vi "DownLoad LTC-20 Table V0.80.vi"(0 "LTC-20 GPIB":refnum<visa-resource-name>, 2 "Sensor Selection":u16(ring) items=["Old MultiSample30T", "New MultiSample Probe (heavy)", "TransmissionProbe 30T", "Double Sample 30T", "SingleSample 30T", "Voigt-6SampleProbe 20T", "Nurmikko30T Top-emission", "Wim MOKE Probe"], 5 "error in (no error)":errorcluster, 9 "Sensor BasePath":path=path "/Optics2mac/Thermometer Calibrations/ Optics") -> (14 "#Tables":i32, 16 "ManyCal?":string, 19 "error out":errorcluster)   [LabVIEW 2019]
uses:
  <vilib>/Utility/file.llb/Read From Spreadsheet File (DBL).vi
panel:
  in  "?":bool
  in  "?":bool
  out "Sensor":string=":CX1050X10903"
  out "Loading:":i32
  out "CalArray":string[](array[string])=["325.000,2.02480,", "320.000,2.02830,", "310.000,2.03560,", "300.000,2.04330,", "290.000,2.05150,", "280.000,2.05960,", "270.000,2.06840,", "260.000,2.07700,", "250.000,2.08660,", "240.000,2.09600,", "230.000,2.10620,", "220.000,2.11640,", "210.000,2.12740,", "200.000,2.13890,", "190.000,2.15060,", "180.000,2.16290,", "170.000,2.17600,", "160.000,2.18960,", "150.000,2.20390,", "140.000,2.21930,", "130.000,2.23510,", "120.000,2.25180,", "110.000,2.26960,", "100.000,2.28870,", "90.000,2.30910,", "80.000,2.33160,", "77.350,2.33790,", "75.000,2.34350,", "70.000,2.35620,", "60.000,2.38390,", "56.000,2.39580,", "54.000,2.40200,", "50.000,2.41500,", "46.000,2.42910,", "44.000,2.43630,", "40.000,2.45170,", "38.000,2.45980,", "36.000,2.46820,", "34.000,2.47700,", "32.000,2.48650,", "30.000,2.49610,", "28.000,2.50610,", "26.000,2.51680,", "24.000,2.52810,", "22.000,2.54030,", "20.000,2.55340,", "19.000,2.56040,", "18.000,2.56750,", "17.000,2.57510,", "16.000,2.58310,", "15.000,2.59170,", "14.000,2.60120,", "13.000,2.61050,", "12.000,2.62100,", "11.000,2.63250,", "10.000,2.64480,", "9.500,2.65150,", "9.000,2.65880,", "8.500,2.66660,", "8.000,2.67440,", "7.500,2.68330,", "7.000,2.69270,", "6.500,2.70230,", "6.000,2.71370,", "5.800,2.71840,", "5.400,2.72870,", "5.000,2.73950,", "4.600,2.75160,", "4.200,2.76480,", "4.000,2.77230,", "3.900,2.77610,", "3.800,2.78000,", "3.700,2.78390,", "3.600,2.78810,", "3.500,2.79240,", "3.400,2.79700,", "3.300,2.80160,", "3.200,2.80650,", "3.100,2.81150,", "3.000,2.81660,", "2.900,2.82200,", "2.800,2.82780,", "2.700,2.83370,", "2.600,2.84000,", "2.500,2.84660,", "2.400,2.85350,", "2.300,2.86120,", "2.200,2.86870,", "2.100,2.87700,", "2.000,2.88560,", "1.900,2.89500,", "1.800,2.90520,", "1.700,2.91630,", "1.600,2.92920,", "1.500,2.94380,", "1.400,2.96020,", "1.300,2.97870,"]
  out "CharMatch":string="SCALT4,2,0,OptCernoxX02158,-1.0,"
  out "TempData":sgl[](array[numeric])=[325.0, 320.0, 310.0, 300.0, 290.0, 280.0, 270.0, 260.0, 250.0, 240.0, 230.0, 220.0, 210.0, 200.0, 190.0, 180.0, 170.0, 160.0, 150.0, 140.0, 130.0, 120.0, 110.0, 100.0, 90.0, 80.0, 77.35, 75.0, 70.0, 60.0, 56.0, 54.0, 50.0, 46.0, 44.0, 40.0, 38.0, 36.0, 34.0, 32.0, 30.0, 28.0, 26.0, 24.0, 22.0, 20.0, 19.0, 18.0, 17.0, 16.0, 15.0, 14.0, 13.0, 12.0, 11.0, 10.0, 9.5, 9.0, 8.5, 8.0, 7.5, 7.0, 6.5, 6.0, 5.8, 5.4, 5.0, 4.6, 4.2, 4.0, 3.9, 3.8, 3.7, 3.6, 3.5, 3.4, 3.3, 3.2, 3.1, 3.0, 2.9, 2.8, 2.7, 2.6, 2.5, 2.4, 2.3, 2.2, 2.1, 2.0, 1.9, 1.8, 1.7, 1.6, 1.5, 1.4, 1.3] format="%.2f"
  out "LogOhms":sgl[](array[numeric])=[2.0248, 2.0283, 2.0356, 2.0433, 2.0515, 2.0596, 2.0684, 2.077, 2.0866, 2.096, 2.1062, 2.1164, 2.1274, 2.1389, 2.1506, 2.1629, 2.176, 2.1896, 2.2039, 2.2193, 2.2351, 2.2518, 2.2696, 2.2887, 2.3091, 2.3316, 2.3379, 2.3435, 2.3562, 2.3839, 2.3958, 2.402, 2.415, 2.4291, 2.4363, 2.4517, 2.4598, 2.4682, 2.477, 2.4865, 2.4961, 2.5061, 2.5168, 2.5281, 2.5403, 2.5534, 2.5604, 2.5675, 2.5751, 2.5831, 2.5917, 2.6012, 2.6105, 2.621, 2.6325, 2.6448, 2.6515, 2.6588, 2.6666, 2.6744, 2.6833, 2.6927, 2.7023, 2.7137, 2.7184, 2.7287, 2.7395, 2.7516, 2.7648, 2.7723, 2.7761, 2.78, 2.7839, 2.7881, 2.7924, 2.797, 2.8016, 2.8065, 2.8115, 2.8166, 2.822, 2.8278, 2.8337, 2.84, 2.8466, 2.8535, 2.8612, 2.8687, 2.877, 2.8856, 2.895, 2.9052, 2.9163, 2.9292, 2.9438, 2.9602, 2.9787] format="%.2f"
  out "Sensor Path":path=path "/Opticsmac/Thermometer Calibrations/ Optics"
  in  "Sensor Array":T1(array[cluster])=[{"Sensor Path"=path "CX1050X10903", "Sensor Info"="Old MultiSample30T"}, {"Sensor Path"=path "CX1050X10904", "Sensor Info"="New MultiSample Probe (heavy)"}, {"Sensor Path"=path "CX1050X10905", "Sensor Info"="TransmissionProbe 30T"}, {"Sensor Path"=path "CX1050X10906", "Sensor Info"="Double Sample 30T"}, {"Sensor Path"=path "", "Sensor Info"="SingleSample 30T"}, {"Sensor Path"=path "", "Sensor Info"="Voigt-6SampleProbe 20T"}, {"Sensor Path"=path "NML-Opt Cernox X04975.cal", "Sensor Info"="Nurmikko30T Top-emission"}, {"Sensor Path"=path "cernox 1010(x01974).rev", "Sensor Info"="Wim MOKE Probe"}]
  # "Tested successfully on S/N 0195"
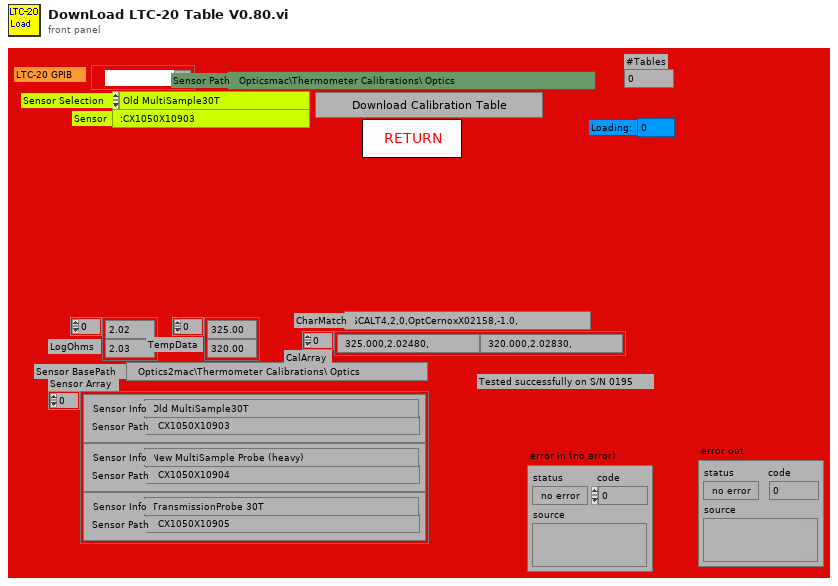
[diagram p1: front panel]
types:
  T1 = cluster{"Sensor Path":path, "Sensor Info":string}[]
  T2 = cluster{"Sensor Path":path, "Sensor Info":string}
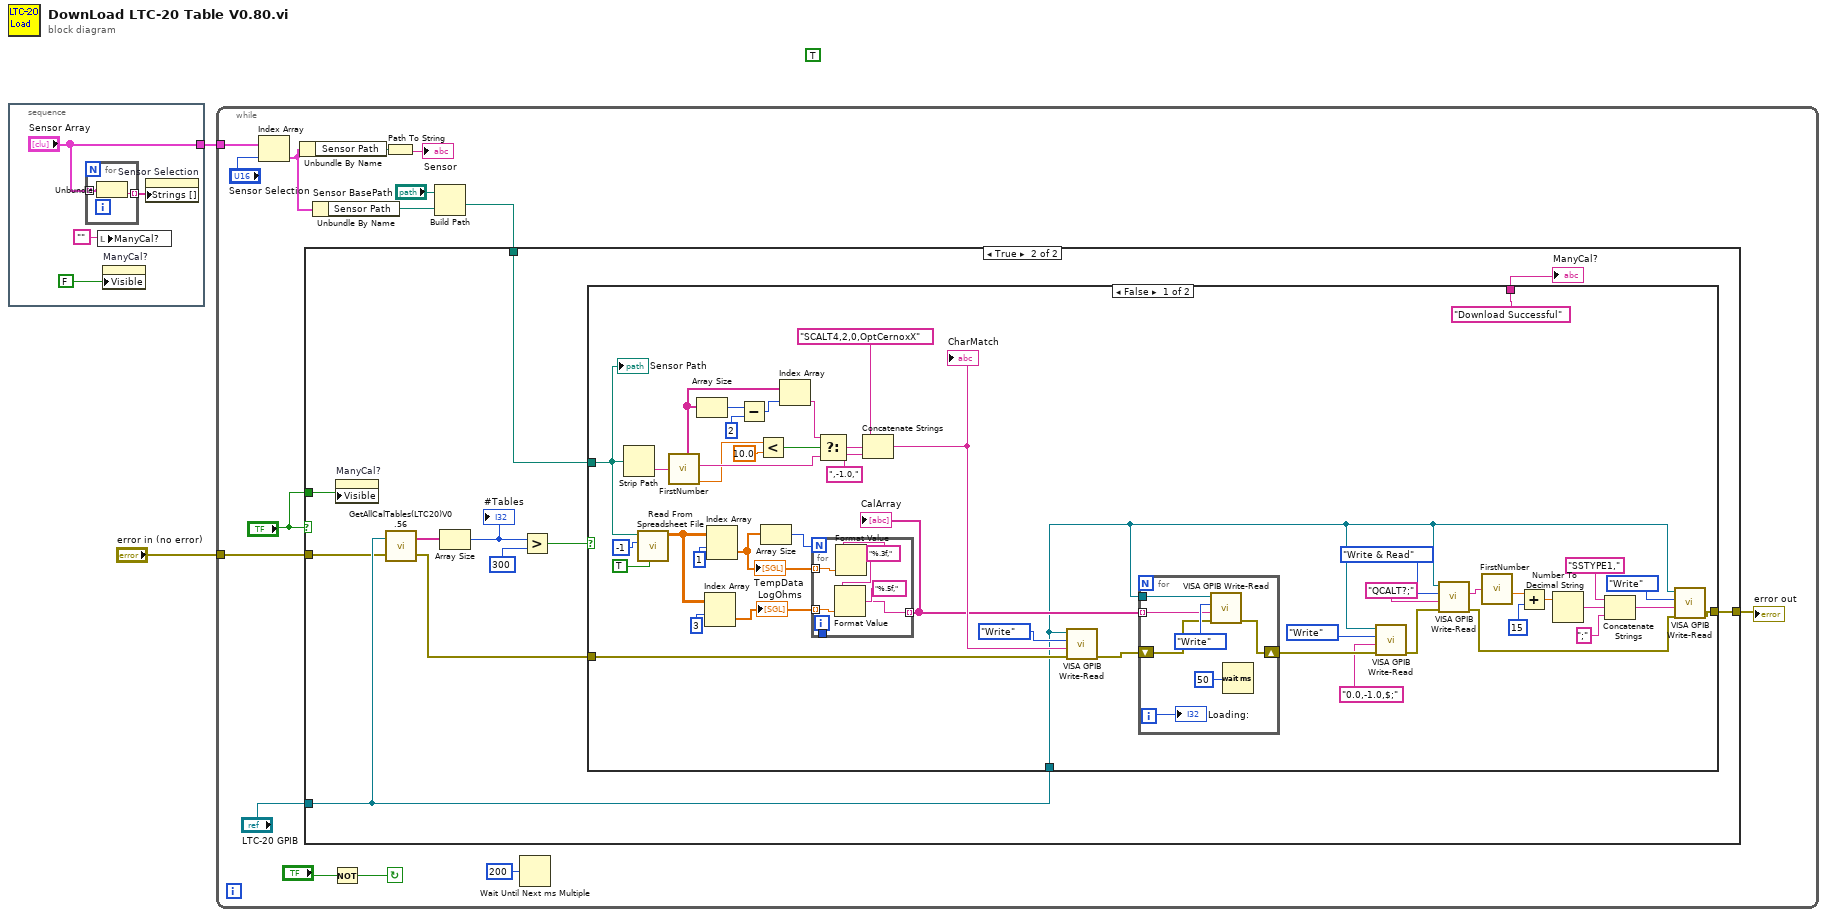
[diagram p0: block diagram]
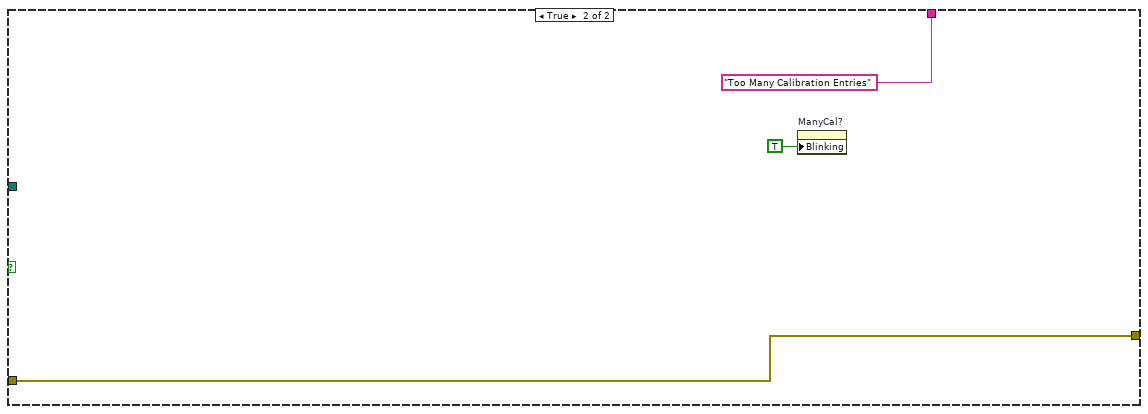
[diagram p3: hidden frame]
diagram:
  (unwired) TRUE
  n1 = stacked-sequence {
    tunnel: ["Sensor Array"] -> w2
    frame #0 {
      n2 = for {
        tunnel: "Sensor Array" -> [w8] mode=indexing
        tunnel: [w7] -> w5 mode=indexing
        n3 = Unbundle(w8) -> ("Sensor Info"=w7:string)  [unwired: 1 out]
      }
      n4 = local write "ManyCal?"("") -> ()
      n5 = property on="ManyCal?" class="Str"("Visible"=FALSE) -> ()  [unwired: 2 in, 2 out]
      n6 = property on="Sensor Selection" class="Ring (strict)"("Strings []"=w5) -> ()  [unwired: 2 in, 2 out]
    }
  }
  n7 = while {
    tunnel: "error in (no error)" -> [w10]
    tunnel: w2 -> [w20]
    stop <- w14 continue-if-true
    n8 = Index Array(array=w20, index="Sensor Selection") -> (element=w19:T2)
    n9 = Unbundle By Name(w19) -> ("Sensor Path"=w22:path)
    n10 = Unbundle By Name(w19) -> ("Sensor Path"=w18:path)
    n11 = Not(x="?") -> (.not. x?=w14:bool)
    n12 = Path To String(path=w22) -> (string=→"Sensor":string)
    n13 = Build Path(base path="Sensor BasePath", name or relative path=w18) -> (appended path=w16:path)
    n14 = case shown="True" "?" {
      tunnel: w16 -> [_ w35]
      tunnel: "LTC-20 GPIB" -> [_ w30]
      tunnel: "?" -> [_ w29]
      tunnel: w10 -> [w24 w27]
      tunnel: [w24 w25] -> w9
      frame False {
      }
      frame True {
        n15 = property on="ManyCal?" class="Str"("Visible"=w29) -> ()  [unwired: 2 in, 2 out]
        n16 = call "GetAllCalTables(LTC20)V0.56.vi"("error in (no error)"=w27, "LTC-20 IEEE"=w30) -> ("error out"=w26:errorcluster, "CalTables"=w34:string[])
        n17 = Array Size(array=w34) -> (size(s)=w32:i32)
        "#Tables" <- w32
        n18 = Greater?(x=w32, y=300) -> (0:w31:bool)
        n19 = case shown="False" w31 {
          tunnel: w35 -> [w69 _]
          tunnel: w30 -> [w36 _]
          tunnel: ["Download Successful" "Too Many Calibration Entries"] -> w28
          tunnel: w26 -> [w55 w96]
          tunnel: [w37 w96] -> w25
          frame False {
            n20 = Strip Path(path=w69) -> (name=w72:string)  [unwired: 1 out]
            n21 = call-poly <vilib>:"Read From Spreadsheet File.vi"("transpose (no:F)"=TRUE, "number of rows (all:-1)"=-1, "file path (dialog if empty)"=w69) -> ("all rows"=w63:dbl[][])  [unwired: 4 in, 4 out]
            n22 = call "FirstNumber.vi"("Input String"=w72) -> ("Number Stings"=w75:string[], 4:"LastNumber"=w81:string, 6:"LastNumber"=w73:ext)  [unwired: 3 out]
            n23 = Array Size(array=w75) -> (size(s)=w77:i32)
            n24 = Index Array(array=w63, index (row)=3) -> (element=w67:dbl[])  [unwired: 1 in]
            "LogOhms" <- w67
            n25 = Index Array(array=w63, index (row)=1) -> (element=w66:dbl[])  [unwired: 1 in]
            "TempData" <- w66
            n26 = Subtract(x=w77, y=2) -> (x-y=w76:i32)
            n27 = Less?(x=w73, y=10.0) -> (x < y?=w79:bool)
            n28 = Array Size(array=w66) -> (size(s)=w68:i32)
            n29 = Index Array(array=w75, index=w76) -> (element=w80:string)
            n30 = for {
              N: w68 -> [_]
              tunnel: w66 -> [w90] mode=indexing
              tunnel: w67 -> [w95] mode=indexing
              tunnel: [w92] -> w58 mode=indexing
              tunnel: [w89] -> _
              i -> [w89]
              n31 = Format Value(format string="%.3f,", value (0)=w90) -> (output string=w91:string)  [unwired: 1 in]
              n32 = Format Value(string ("")=w91, format string="%.5f,", value (0)=w95) -> (output string=w92:string)
            }
            "CalArray" <- w58
            n33 = Select(t=w80, s=w79, f=w81) -> (s? t:f=w59:string)
            n34 = Concatenate Strings("SCALT4,2,0,OptCernoxX", w59, ",-1.0,") -> (w62:string)
            "CharMatch" <- w62
            n35 = call "VISA GPIB Write-Read.vi"("error in (no error)"=w55, "Command"=w62, "Action"=enum16{"Write", "Read", "Write & Read"}."Write", "VISA resource name"=w36) -> ("error out"=w54:errorcluster)  [unwired: 4 in, 3 out]
            n36 = for {
              tunnel: w36 -> [w82]
              tunnel: w58 -> [w85] mode=indexing
              shift-right: [w83] -> w53
              shift-left: w54 -> [w84]
              i -> [w88]
              n37 = call "VISA GPIB Write-Read.vi"("error in (no error)"=w84, "Command"=w85, "Action"=enum16{"Write", "Read", "Write & Read"}."Write", "VISA resource name"=w82) -> ("error out"=w83:errorcluster)  [unwired: 4 in, 3 out]
              n38 = Wait (ms)(milliseconds to wait=u32 50) -> ()  [unwired: 1 out]
              "Loading:" <- w88
            }
            n39 = call "VISA GPIB Write-Read.vi"("error in (no error)"=w53, "Command"="0.0,-1.0,$;", "Action"=enum16{"Write", "Read", "Write & Read"}."Write", "VISA resource name"=w36) -> ("error out"=w52:errorcluster)  [unwired: 4 in, 3 out]
            n40 = call "VISA GPIB Write-Read.vi"("error in (no error)"=w52, "Command"="QCALT?;", "Action"=enum16{"Write", "Read", "Write & Read"}."Write & Read", "VISA resource name"=w36) -> ("error out"=w38:errorcluster, "String Returned"=w41:string)  [unwired: 4 in, 2 out]
            n41 = call "FirstNumber.vi"("Input String"=w41) -> ("FirstNumber"=w47:ext)  [unwired: 5 out]
            n42 = Add(x=w47, y=15) -> (x+y=w48:ext)
            n43 = Number To Decimal String(number=w48) -> (decimal integer string=w49:string)  [unwired: 1 in]
            n44 = Concatenate Strings("SSTYPE1,", w49, ";") -> (w40:string)
            n45 = call "VISA GPIB Write-Read.vi"("error in (no error)"=w38, "Command"=w40, "Action"=enum16{"Write", "Read", "Write & Read"}."Write", "VISA resource name"=w36) -> ("error out"=w37:errorcluster)  [unwired: 4 in, 3 out]
            "Sensor Path" <- w69
          }
          frame True {
            n46 = property on="ManyCal?" class="Str"("Blinking"=TRUE) -> ()  [unwired: 2 in, 2 out]
          }
        }
        "ManyCal?" <- w28
      }
    }
    "error out" <- w9
    n47 = Wait Until Next ms Multiple(millisecond multiple=u32 200) -> ()  [unwired: 1 out]
  }
